vi "WinHostTocRIO.vi"() -> ()   [LabVIEW 2013]
uses:
  <vilib>/userdefined/High Color/nirio_resource_hc.ctl
  <vilib>/nisyscfg/Find Hardware.vi
  <vilib>/nisyscfg/Close (System).vi
  <vilib>/FPGAPlugInAG/NI 9159/niLvFpga_Open_NI 9159.vi
  <vilib>/rvi/interface/common/dynamic/niFpgaDynamicAddResources.vi
  <vilib>/rvi/interface/common/niFpgaWaitOnOcc.vi
  <vilib>/Utility/error.llb/Error Cluster From Error Code.vi
  <vilib>/FPGAPlugInAG/Dynamic/niLvFpga_Reset_Dynamic.vi
  <vilib>/FPGAPlugInAG/Dynamic/niLvFpga_Run_Dynamic.vi
  <vilib>/rvi/errors/niLvFpgaAdjustHostInterfaceError.vi
  <vilib>/FPGAPlugInAG/Dynamic/niLvFpga_Close_Dynamic.vi
  <vilib>/rvi/interface/nirviOpenFPGA/nirviOpenFPGA.xnode
  FPGA Bitfiles/cRIO9159_cRIODAQDMA_v1_1.lvbitx
  <vilib>/rvi/interface/nirviMethod/nirviMethod.xnode
  <vilib>/rvi/interface/nirviReadWriteControl/nirviReadWriteControl.xnode
  <vilib>/rvi/interface/nirviCloseFPGA/nirviCloseFPGA.xnode
  <vilib>/rvi/interface/Simulation/niFpgaSimulationCallBeginRW.vi
  <vilib>/rvi/errors/niLvFpgaMergeErrorWithErrorCode.vi
  <vilib>/FPGAPlugInAG/Dynamic/niLvFpga_ReadFifo_Dynamic.vi
  NiFpgaLv.dll
  <vilib>/nisyscfg/nisyscfg.lvlib
  <resource>/objmgr/nisysapi.rc
  <vilib>/FPGAPlugInAG/Dynamic/niLvFpga_ConfigureFifo_Dynamic.vi
  <vilib>/FPGAPlugInAG/Dynamic/niLvFpga_StartFifo_Dynamic.vi
  <vilib>/FPGAPlugInAG/Dynamic/niLvFpga_StopFifo_Dynamic.vi
panel:
  in  "stop":bool
  out "resource name":T1
  out "Resource":string="RIO0"
  out "resources out":refnum<k20>[](array[refnum])
  out "Waveform Graph":waveform(dbl)[](graph)
  out "error out":errorcluster
  out "Elements Remaining 3":u32
  out "Elements Remaining 2":u32
  in  "Tab Control":T2(tab)
  out "FPGAVIversion":u8[](array[numeric])=[1, 0]
  out "InsertedIOModulesID":u16[](array[numeric]) format="%x"
  out "InitDone":bool
  out "cRIOModulesOK":bool
  in  "DebugMode":bool
  out "DevQualityStatus":u8
  out "DeviceTemp":sgl format="%#1.2f"
  in  "DAQStartStop":bool
  out "DevProfile":u8
  out "Fref":u32
  out "DMATtoHOSTNCh":u16[](array[numeric])=[2]
  out "DMATtoHOSTFrameType":u8[](array[numeric])
  out "DMATtoHOSTSampleSize":u8[](array[numeric])=[4]
  out "DMATtoHOSTBlockNWords":u16[](array[numeric])=[128]
  out "DMATtoHOSTSamplingRate0":u16=1
  out "Elements Remaining":u32
  out "*(type *) &x":i32[](array[numeric])=[-730742, -4984294, -731430, -7767672, -730742, -9796516, -730053, -10862915, -730742, -10864292, -730053, -9799269, -730053, -7779375, -730742, -4991867, -730053, -1712809, -730742, 1728033, -730053, 5007779, -730742, 7793223, -730742, 9820002, -731430, 10887778, -730053, 10889843, -730742, 9825509, -731430, 7804238, -730742, 5014664, -730742, 1735606, -730053, -1705236, -730742, -4985671, -730053, -7766983, -731430, -9796516, -730053, -10861538, -731430, -10864292, -731430, -9799269, -729365, -7777999, -730742, -4991867, -731430, -1712809, -730053, 1727345, -730053, 5007779, -730053, 7791846, -730742, 9820690, -730742, 10887089, -732119, 10889843, -730742, 9824821, -730742, 7804238, -730742, 5013287, -730742, 1734229, -730053, -1705236, -730053, -4984982, -730053, -7766983, -730742, -9796516, -730053, -10862227, -730053, -10863604, -730742, -9799269, -730742, -7780064, -730053, -4991178, -731430, -1713497, -730742, 1726656, -730742, 5007091, -732119, 7792535, -730053, 9820002, -730742, 10887778, -730053, 10887089, -730053, 9824132, -730053, 7804238, -730742, 5014664, -730742, 1734918, -730742, -1705236, -732119, -4983605, -730742, -7766983, -730742, -9795827, -730053, -10862227, -730053, -10864292, -730742, -9799269, -730742, -7778687, -730742, -4990490, -730053, -1713497, -730742, 1728033, -731430, 5007779, -730742, 7791846, -731430, 9820690, -730053, 10887089, -731430, 10888466, -731430, 9824821, -730742, 7804238, -730053, 5013975, -730053, 1736295, -730053, -1704547, -732119, -4983605, -731430, -7766295, -730053, -9795139, -730742, -10861538, -730742, -10862915, -730053, -9798581, -730742, -7778687, -730742, -4991178, -731430, -1712809, -730742, 1725968, -731430, 5007779, -730053, 7791158, -732119, 9820002, -730742, 10887089, -730742, 10888466, -731430, 9824132, -730053, 7805615, -730742, 5015352, -730742, 1736295, -730742, -1704547, -730742, -4983605, -730742, -7766983, -729365, -9795827, -731430, -10862227, -730742, -10863604, -730053, -9800646, -730053, -7779375, -731430, -4991867, -731430, -1712809, -730053, 1726656, -731430, 5007091, -729365, 7792535, -730742, 9820690, -731430, 10887778, -731430, 10888466, -730742, 9824132, -730742, 7804927, -730742, 5014664, -731430, 1736295, -731430, -1702482, -730742, -4983605, -730742, -7766295, -730742, -9795139, -730053, -10862227, -730742, -10864292, -730742, -9799269, -730053, -7780752, -730742, -4992555] format="%x"
  out "Array":fxp<+/-,26,5>[](array[numeric])=[-0.34844493865966797, -2.3766965866088867, -0.3487730026245117, -3.7039146423339844, -0.34844493865966797, -4.671342849731445, -0.348116397857666, -5.1798415184021, -0.34844493865966797, -5.180498123168945, -0.348116397857666, -4.6726555824279785, -0.348116397857666, -3.7094950675964355, -0.34844493865966797, -2.380307674407959, -0.348116397857666, -0.8167309761047363, -0.34844493865966797, 0.8239903450012207, -0.348116397857666, 2.387895107269287, -0.34844493865966797, 3.7160983085632324, -0.34844493865966797, 4.682541847229004, -0.3487730026245117, 5.191697120666504, -0.348116397857666, 5.192681789398193, -0.34844493865966797, 4.6851677894592285, -0.3487730026245117, 3.72135066986084, -0.34844493865966797, 2.3911781311035156, -0.34844493865966797, 0.827601432800293, -0.348116397857666, -0.8131198883056641, -0.34844493865966797, -2.3773531913757324, -0.348116397857666, -3.7035861015319824, -0.3487730026245117, -4.671342849731445, -0.348116397857666, -5.179184913635254, -0.3487730026245117, -5.180498123168945, -0.3487730026245117, -4.6726555824279785, -0.34778833389282227, -3.708838939666748, -0.34844493865966797, -2.380307674407959, -0.3487730026245117, -0.8167309761047363, -0.348116397857666, 0.823662281036377, -0.348116397857666, 2.387895107269287, -0.348116397857666, 3.7154417037963867, -0.34844493865966797, 4.682869911193848, -0.34844493865966797, 5.191368579864502, -0.34910154342651367, 5.192681789398193, -0.34844493865966797, 4.684839725494385, -0.34844493865966797, 3.72135066986084, -0.34844493865966797, 2.39052152633667, -0.34844493865966797, 0.8269448280334473, -0.348116397857666, -0.8131198883056641, -0.348116397857666, -2.3770246505737305, -0.348116397857666, -3.7035861015319824, -0.34844493865966797, -4.671342849731445, -0.348116397857666, -5.179513454437256, -0.348116397857666, -5.180170059204102, -0.34844493865966797, -4.6726555824279785, -0.34844493865966797, -3.7098236083984375, -0.348116397857666, -2.379979133605957, -0.3487730026245117, -0.8170590400695801, -0.34844493865966797, 0.823333740234375, -0.34844493865966797, 2.3875670433044434, -0.34910154342651367, 3.7157702445983887, -0.348116397857666, 4.682541847229004, -0.34844493865966797, 5.191697120666504, -0.348116397857666, 5.191368579864502, -0.348116397857666, 4.684511184692383, -0.348116397857666, 3.72135066986084, -0.34844493865966797, 2.3911781311035156, -0.34844493865966797, 0.8272733688354492, -0.34844493865966797, -0.8131198883056641, -0.34910154342651367, -2.3763680458068848, -0.34844493865966797, -3.7035861015319824, -0.34844493865966797, -4.671014308929443, -0.348116397857666, -5.179513454437256, -0.348116397857666, -5.180498123168945, -0.34844493865966797, -4.6726555824279785, -0.34844493865966797, -3.709167003631592, -0.34844493865966797, -2.3796510696411133, -0.348116397857666, -0.8170590400695801, -0.34844493865966797, 0.8239903450012207, -0.3487730026245117, 2.387895107269287, -0.34844493865966797, 3.7154417037963867, -0.3487730026245117, 4.682869911193848, -0.348116397857666, 5.191368579864502, -0.3487730026245117, 5.192025184631348, -0.3487730026245117, 4.684839725494385, -0.34844493865966797, 3.72135066986084, -0.348116397857666, 2.3908495903015137, -0.348116397857666, 0.8279299736022949, -0.348116397857666, -0.8127913475036621, -0.34910154342651367, -2.3763680458068848, -0.3487730026245117, -3.7032580375671387, -0.348116397857666, -4.6706862449646, -0.34844493865966797, -5.179184913635254, -0.34844493865966797, -5.1798415184021, -0.348116397857666, -4.672327518463135, -0.34844493865966797, -3.709167003631592, -0.34844493865966797, -2.379979133605957, -0.3487730026245117, -0.8167309761047363, -0.34844493865966797, 0.8230056762695312, -0.3487730026245117, 2.387895107269287, -0.348116397857666, 3.715113639831543, -0.34910154342651367, 4.682541847229004, -0.34844493865966797, 5.191368579864502, -0.34844493865966797, 5.192025184631348, -0.3487730026245117, 4.684511184692383, -0.348116397857666, 3.7220072746276855, -0.34844493865966797, 2.3915061950683594, -0.34844493865966797, 0.8279299736022949, -0.34844493865966797, -0.8127913475036621, -0.34844493865966797, -2.3763680458068848, -0.34844493865966797, -3.7035861015319824, -0.34778833389282227, -4.671014308929443, -0.3487730026245117, -5.179513454437256, -0.34844493865966797, -5.180170059204102, -0.348116397857666, -4.673312187194824, -0.348116397857666, -3.7094950675964355, -0.3487730026245117, -2.380307674407959, -0.3487730026245117, -0.8167309761047363, -0.348116397857666, 0.823333740234375, -0.3487730026245117, 2.3875670433044434, -0.34778833389282227, 3.7157702445983887, -0.34844493865966797, 4.682869911193848, -0.3487730026245117, 5.191697120666504, -0.3487730026245117, 5.192025184631348, -0.34844493865966797, 4.684511184692383, -0.34844493865966797, 3.721679210662842, -0.34844493865966797, 2.3911781311035156, -0.3487730026245117, 0.8279299736022949, -0.3487730026245117, -0.8118066787719727, -0.34844493865966797, -2.3763680458068848, -0.34844493865966797, -3.7032580375671387, -0.34844493865966797, -4.6706862449646, -0.348116397857666, -5.179513454437256, -0.34844493865966797, -5.180498123168945, -0.34844493865966797, -4.6726555824279785, -0.348116397857666, -3.7101516723632812, -0.34844493865966797, -2.3806357383728027]
  out "Data":u64[](array[numeric])=[18443605565007720986, 18443602610067437960, 18443605565002908764, 18443608524234309309, 18443605565001840988, 18443608524235372955, 18443608524237392849, 18443605565007713413, 18443608524243459415, 18443605560719466017, 18443608519955212707, 18443605560725531207, 18443605560727557986, 18443602605791126114, 18443608519961094771, 18443605560727563493, 18443602605788042574, 18443605560722752648, 18443605560719473590, 18443608524243466988, 18443605565007719609, 18443608524237405241, 18443602610065409116, 18443608524234310686, 18443602610064341340, 18443602610065406363, 18443611479174893873, 18443605565007713413, 18443602610073492823, 18443608519951932273, 18443608519955212707, 18443608519957996774, 18443605560727558674, 18443605560728625073, 18443599646558661235, 18443605560727562805, 18443605560725542222, 18443605560722751271, 18443605560719472213, 18443608524243466988, 18443608524240187242, 18443608524237405241, 18443605565002908764, 18443608524234309997, 18443608524234308620, 18443605565002906011, 18443605565004925216, 18443608524240181046, 18443602610073492135, 18443605560719464640, 18443605560722745075, 18443599646555563927, 18443608519960024930, 18443605560728625762, 18443608519961092017, 18443608519960029060, 18443608519958009166, 18443605560722752648, 18443605560719472902, 18443605565011000044, 18443599650837755083, 18443605565004938297, 18443605565002909453, 18443608524234309997, 18443608524234307932, 18443605565002906011, 18443605565004926593, 18443605565007714790, 18443608524243458727, 18443605560719466017, 18443602605785246115, 18443605560725529830, 18443602605790059026, 18443608519961092017, 18443602605791126802, 18443602605790063157, 18443605560725542222, 18443608519955218903, 18443608519951941223, 18443608524243467677, 18443599650837755083, 18443602610067439337, 18443608524235377085, 18443605565001843742, 18443605565001842365, 18443608524235373643, 18443605565004926593, 18443605565007714102, 18443602610073492823, 18443605560719463952, 18443602605785246115, 18443608519957996086, 18443599646557591394, 18443605560728625073, 18443605560728626450, 18443602605790062468, 18443608519958010543, 18443605560722753336, 18443605560719474279, 18443605565011000733, 18443605565007721675, 18443605565004938297, 18443611479172876045, 18443602610064343405, 18443605565001841676, 18443608524235371578, 18443608524237392849, 18443602610070213765, 18443602610073492823, 18443608519951931584, 18443602605785245427, 18443611474895497111, 18443605560727558674, 18443602605791126114, 18443602605791126802, 18443605560727562116, 18443605560725542911, 18443605560722752648, 18443602605781974631, 18443602610073503150, 18443605565007721675, 18443605565004938985, 18443605565002910141, 18443608524234309997, 18443605565001840988, 18443605565002906011, 18443608524237391472, 18443605565007712725]
  in  "AO0":fxp<+/-,20,5>
  in  "AO1":fxp<+/-,20,5>
  in  "SGSignalType0":u8=1 max=3
  in  "SGPhase0":u32
  out "SGAmp0":u16
  in  "SGFreq0":sgl=50.0
  in  "SGAmp0":fxp<+/-,20,5>
  in  "SGUpdateRate0":u32=50
  out "AI1":fxp<+/-,26,5>
  out "AI0":fxp<+/-,26,5>
  in  "AOEnable0":bool
  in  "AOEnable1":bool
  out "AI2":fxp<+/-,26,5>
  in  "AO2":fxp<+/-,20,5>
  in  "AOEnable2":bool
  out "SGFref0":u32
  in  "Desired Sampling Rate":dbl=1000.0 max=1000.0
  out "SamplingRate":dbl
  in  "DO0":bool
  in  "DO1":bool
  in  "DO2":bool
  in  "auxDO1":bool
  out "DI0":bool
  out "DI1":bool
  out "DI2":bool
  out "auxDI1":bool
  out "Numeric":i32
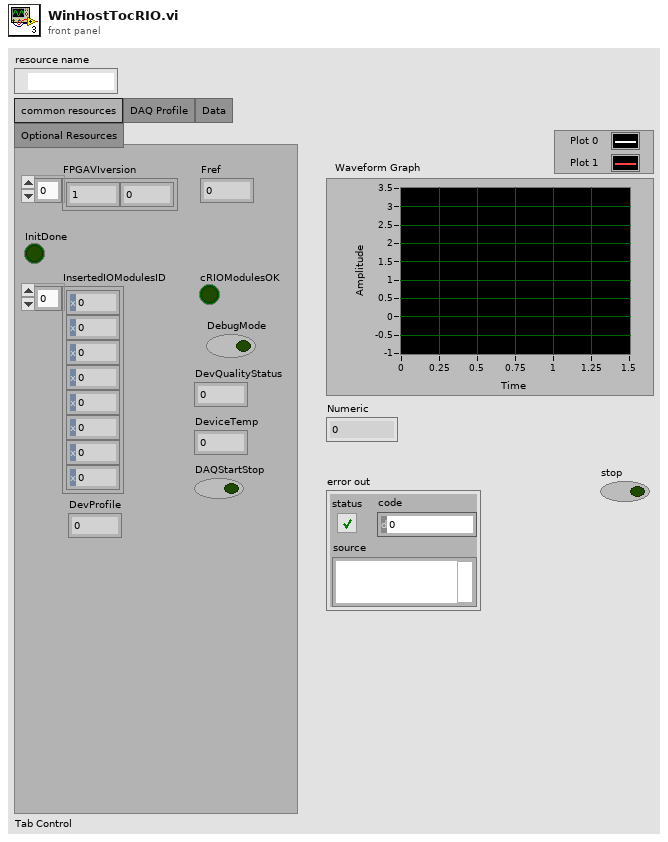
[diagram p1: front panel]
types:
  T1 = typedef "nirio_resource_hc.ctl" = tag
  T2 = enum32{"common resources", "DAQ Profile", "Data", "Optional Resources"}
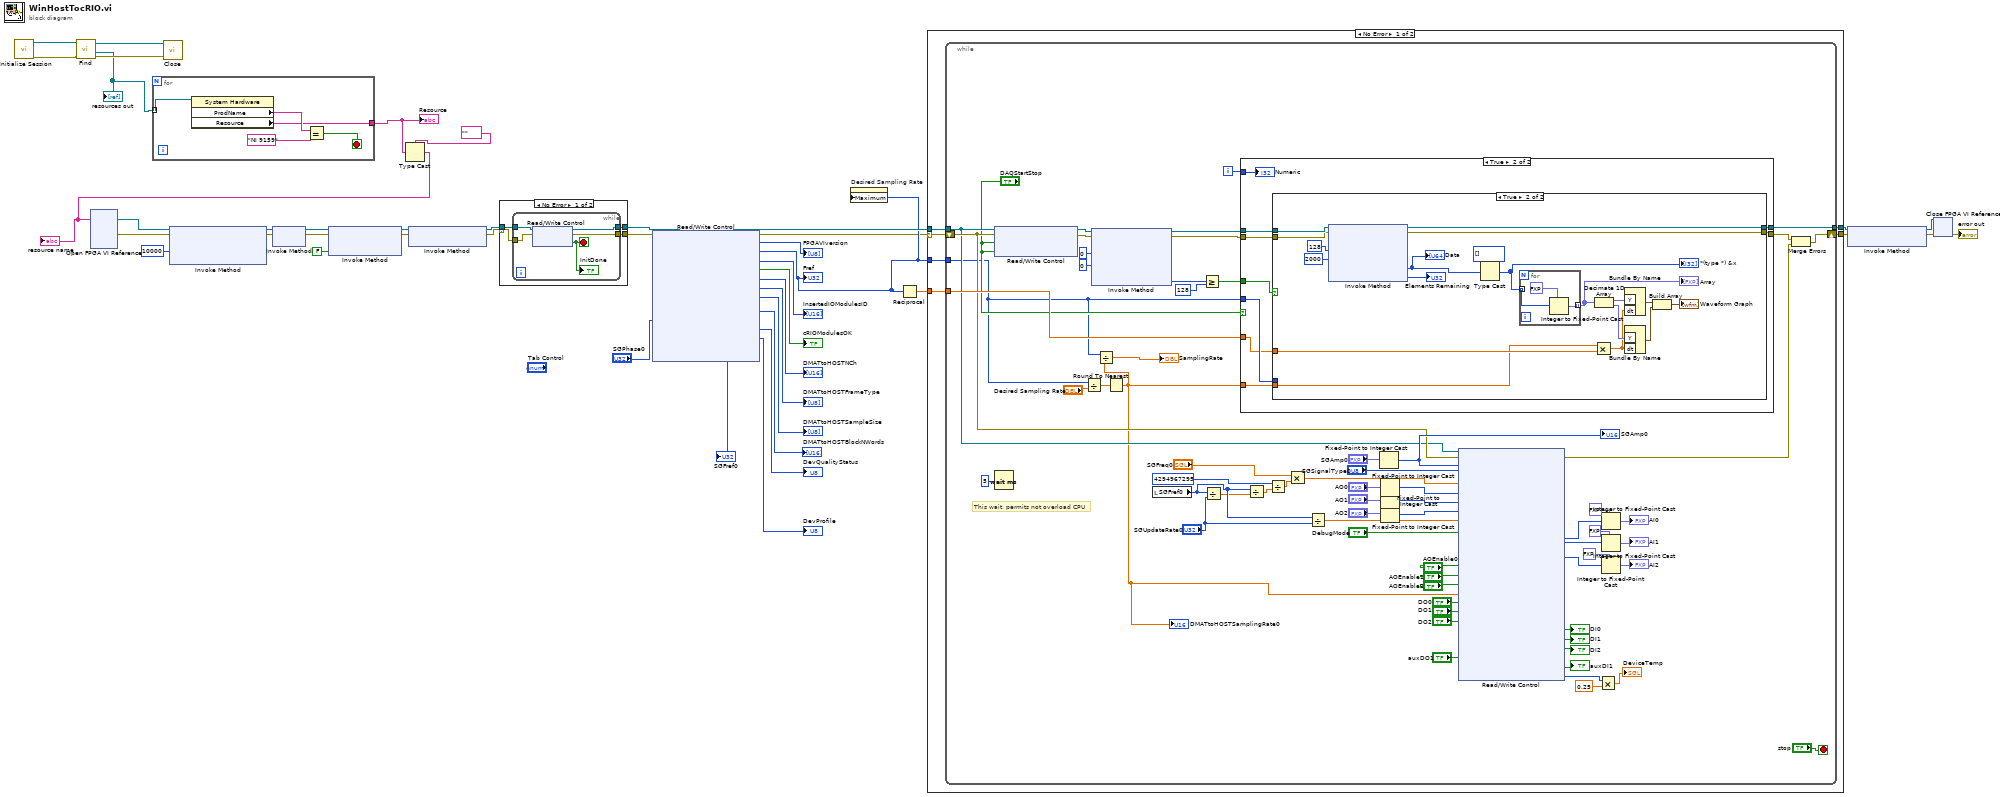
[diagram p0: block diagram]
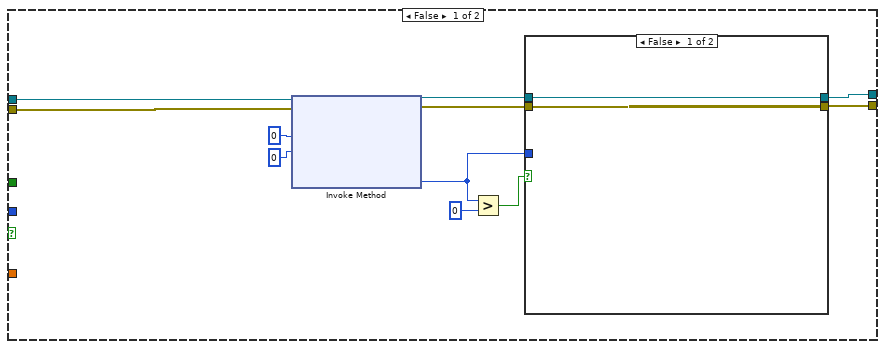
[diagram p2: hidden frame]
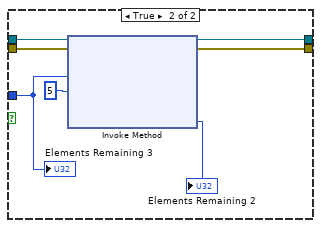
[diagram p3: hidden frame]
diagram:
  n1 = call <vilib>:"Initialize Session.vi"() -> ("error out"=w7:errorcluster, "session out"=w8:refnum<k21>)  [unwired: 10 in]
  n2 = call-poly <vilib>:"Find.vi"("error in (no error)"=w7, "session in"=w8) -> ("error out"=w5:errorcluster, "resources out"=w4:refnum<k20>[], "session out"=w6:refnum<k21>)  [unwired: 6 in, 1 out]
  "resources out" <- w4
  n3 = for {
    tunnel: w4 -> [w47] mode=indexing
    tunnel: [w43] -> w3
    stop <- w44 stop-if-true
    n4 = property class="System Hardware"(reference=w47) -> ("ProdName"=w45:string, "Resource"=w43:string)  [unwired: 1 in, 2 out]
    n5 = Equal?(x=w45, y="NI 9159") -> (x = y?=w44:bool)
  }
  "Resource" <- w3
  n6 = call-poly <vilib>:"Close.vi"("error in (no error)"=w5, "session in"=w6) -> ()  [unwired: 9 in, 1 out]
  n7 = Type Cast(type=T1 "" ("resource name 2"), x=w3) -> (*(type *) &x=w1:T1)
  "resource name" <- w1
  n8 = xnode "Open FPGA VI Reference"("resource name"=w1) -> ("FPGA VI Reference Out"=w30:refnum<k20>, "error out"=w29:errorcluster)  [unwired: 1 in]
  n9 = xnode "Invoke Method"("FPGA VI Reference In"=w30, "error in"=w29, "Requested Depth"=u32 10000) -> ("FPGA VI Reference Out"=w28:refnum<k20>, "error out"=w27:errorcluster)  [unwired: 1 out]
  n10 = xnode "Invoke Method"("FPGA VI Reference In"=w28, "error in"=w27) -> ("FPGA VI Reference Out"=w42:refnum<k20>, "error out"=w41:errorcluster)
  n11 = xnode "Invoke Method"("FPGA VI Reference In"=w42, "error in"=w41, "Wait Until Done (F)"=FALSE) -> ("FPGA VI Reference Out"=w25:refnum<k20>, "error out"=w24:errorcluster)
  n12 = xnode "Invoke Method"("FPGA VI Reference In"=w25, "error in"=w24) -> ("FPGA VI Reference Out"=w23:refnum<k20>, "error out"=w11:errorcluster)
  n13 = case shown="No Error" w11 {
    selector: w11 -> [w48 w58]
    tunnel: [w51 w57] -> w38
    tunnel: [w50 w58] -> w37
    tunnel: w23 -> [w49 w57]
    frame No Error {
      n14 = while {
        tunnel: w49 -> [w56]
        tunnel: [w54] -> w51
        tunnel: [w53] -> w50
        tunnel: w48 -> [w52]
        stop <- w55 stop-if-true
        n15 = xnode "Read/Write Control"("FPGA VI Reference In"=w56, "error in"=w52) -> ("FPGA VI Reference Out"=w54:refnum<k20>, "error out"=w53:errorcluster, "InitDone"=w55:bool)
        "InitDone" <- w55
      }
    }
    frame Error {
    }
  }
  n16 = xnode "Read/Write Control"("FPGA VI Reference In"=w38, "error in"=w37, "SGPhase0"="SGPhase0") -> ("FPGA VI Reference Out"=w31:refnum<k20>, "error out"=w10:errorcluster, "FPGAVIversion"=→"FPGAVIversion":u8[], "Fref"=w13:u32, "InsertedIOModulesID"=→"InsertedIOModulesID":u16[], "cRIOModulesOK"=→"cRIOModulesOK":bool, "DMATtoHOSTNCh"=→"DMATtoHOSTNCh":u16[], "DMATtoHOSTFrameType"=→"DMATtoHOSTFrameType":u8[], "DMATtoHOSTSampleSize"=→"DMATtoHOSTSampleSize":u8[], "DMATtoHOSTBlockNWords"=→"DMATtoHOSTBlockNWords":u16[], "DevQualityStatus"=→"DevQualityStatus":u8, "DevProfile"=→"DevProfile":u8, "SGFref0"=→"SGFref0":u32)  [unwired: 1 in]
  "Fref" <- w13
  n17 = property on="Desired Sampling Rate" class="DigNum (strict)"("Maximum"=w13) -> ()  [unwired: 2 in, 2 out]
  n18 = Reciprocal(x=w13) -> (1/x=w14:dbl)
  n19 = case shown="No Error" w10 {
    selector: w10 -> [w59 w186]
    tunnel: w31 -> [w64 w185]
    tunnel: [w63 w185] -> w22
    tunnel: [w62 w186] -> w21
    tunnel: w14 -> [w61 _]
    tunnel: w13 -> [w60 _]
    frame No Error {
      n20 = while {
        tunnel: w64 -> [w79]
        tunnel: [w130] -> w63
        tunnel: w61 -> [w128]
        tunnel: w60 -> [w66]
        shift-right: [w81] -> w62
        shift-left: w59 -> [w80]
        i -> [w129]
        stop <- "stop" stop-if-true
        # "This wait, permits not overload CPU"
        n21 = xnode "Read/Write Control"("FPGA VI Reference In"=w79, "error in"=w80, "DMATtoHOSTEnable0"="DAQStartStop", "DAQStartStop"="DAQStartStop") -> ("FPGA VI Reference Out"=w77:refnum<k20>, "error out"=w76:errorcluster)
        n22 = Wait (ms)(milliseconds to wait=u32 5) -> ()  [unwired: 1 out]
        n23 = Divide(x=w66, y="Desired Sampling Rate") -> (x/y=w85:dbl)
        n24 = xnode "Invoke Method"("FPGA VI Reference In"=w77, "error in"=w76, "Number of Elements"=u32 0, "Timeout (ms)"=0) -> ("FPGA VI Reference Out"=w72:refnum<k20>, "error out"=w71:errorcluster, "Elements Remaining"=w75:u32)  [unwired: 1 out]
        n25 = Round To Nearest(number=w85) -> (nearest integer value=w65:dbl)
        "DMATtoHOSTSamplingRate0" <- w65
        n26 = Divide(x=w66, y=w65) -> (x/y=→"SamplingRate":dbl)
        n27 = local read "SGFref0"() -> (w116:u32)
        n28 = Greater Or Equal?(x=w75, y=u32 128) -> (x >= y?=w70:bool)
        n29 = Divide(x=w116, y="SGUpdateRate0") -> (x/y=w105:dbl)
        n30 = case shown="True" "DAQStartStop" {
          tunnel: [w138 w152] -> w130
          tunnel: [w137 w156] -> w83
          tunnel: w129 -> [_ w160]
          tunnel: w128 -> [_ w158]
          tunnel: w66 -> [_ w159]
          tunnel: w65 -> [_ w157]
          tunnel: w72 -> [w133 w154]
          tunnel: w71 -> [w132 w153]
          tunnel: w70 -> [_ w155]
          frame False {
            n31 = xnode "Invoke Method"("FPGA VI Reference In"=w133, "error in"=w132, "Number of Elements"=u32 0, "Timeout (ms)"=0) -> ("FPGA VI Reference Out"=w140:refnum<k20>, "error out"=w139:errorcluster, "Elements Remaining"=w134:u32)  [unwired: 1 out]
            n32 = Greater?(x=w134, y=u32 0) -> (0:w135:bool)
            n33 = case shown="False" w135 {
              tunnel: w140 -> [w144 w151]
              tunnel: w139 -> [w143 w150]
              tunnel: [w144 w147] -> w138
              tunnel: [w143 w146] -> w137
              tunnel: w134 -> [_ w145]
              frame False {
              }
              frame True {
                n34 = xnode "Invoke Method"("FPGA VI Reference In"=w151, "error in"=w150, "Number of Elements"=w145, "Timeout (ms)"=5) -> ("FPGA VI Reference Out"=w147:refnum<k20>, "error out"=w146:errorcluster, "Elements Remaining"=→"Elements Remaining 2":u32)  [unwired: 1 out]
                "Elements Remaining 3" <- w145
              }
            }
          }
          frame True {
            n35 = case shown="True" w155 {
              tunnel: w159 -> [_ _]
              tunnel: w158 -> [_ w169]
              tunnel: w157 -> [_ w168]
              tunnel: [w161 w166] -> w156
              tunnel: w154 -> [w162 w165]
              tunnel: w153 -> [w161 w164]
              tunnel: [w162 w163] -> w152
              frame False {
              }
              frame True {
                n36 = xnode "Invoke Method"("FPGA VI Reference In"=w165, "error in"=w164, "Number of Elements"=u32 128, "Timeout (ms)"=2000) -> ("FPGA VI Reference Out"=w163:refnum<k20>, "error out"=w166:errorcluster, "Data"=w179:u64[], "Elements Remaining"=→"Elements Remaining":u32)
                "Data" <- w179
                n37 = Type Cast(type=i32[] [], x=w179) -> (*(type *) &x=w177:i32[])
                "*(type *) &x" <- w177
                n38 = for {
                  tunnel: w177 -> [w184] mode=indexing
                  tunnel: [w183] -> w176 mode=indexing
                  n39 = Integer to Fixed-Point Cast(fixed-point type=fxp<+/-,26,5> 0.0, integer=w184) -> (fixed-point=w183:fxp<+/-,26,5>)
                }
                "Array" <- w176
                n40 = Multiply(x=w168, y=w169) -> (x*y=w171:dbl)
                n41 = Decimate 1D Array(w176) -> (w175:fxp<+/-,26,5>[], w173:fxp<+/-,26,5>[])
                n42 = Bundle By Name("Y"=w175, "dt"=w171) -> (w174:waveform(dbl))  [unwired: 1 in]
                n43 = Bundle By Name("Y"=w173, "dt"=w171) -> (w172:waveform(dbl))  [unwired: 1 in]
                n44 = Build Array(w174, w172) -> (→"Waveform Graph":waveform(dbl)[])
              }
            }
            "Numeric" <- w160
          }
        }
        n45 = Divide(x=w116, y=w105) -> (x/y=w107:dbl)
        n46 = Divide(x=i64 4294967295, y=w107) -> (x/y=w108:dbl)
        n47 = Multiply(x="SGFreq0", y=w108) -> (x*y=w109:dbl)
        n48 = Divide(x=w116, y="SGUpdateRate0") -> (x/y=w94:dbl)
        n49 = Fixed-Point to Integer Cast(1:"SGAmp0") -> (0:w93:i32)
        "SGAmp0" <- w93
        n50 = Fixed-Point to Integer Cast(1:"AO0") -> (0:w89:i32)
        n51 = Fixed-Point to Integer Cast(1:"AO1") -> (0:w91:i32)
        n52 = Fixed-Point to Integer Cast(1:"AO2") -> (0:w115:i32)
        n53 = xnode "Read/Write Control"("FPGA VI Reference In"=w79, "error in"=w80, "SGAmp0"=w93, "SGSignalType0"="SGSignalType0", "SGFreq0"=w109, "AO0"=w89, "AO1"=w91, "AO2"=w115, "SGUpdateRate0"=w94, "DebugMode"="DebugMode", "AOEnable0"="AOEnable0", "AOEnable1"="AOEnable1", "AOEnable2"="AOEnable2", "DMATtoHOSTSamplingRate0"=w65, "DO0"="DO0", "DO1"="DO1", "DO2"="DO2", "auxDO0"="auxDO1") -> ("error out"=w82:errorcluster, "AI0"=w111:i32, "AI1"=w113:i32, "AI2"=w114:i32, "DI0"=→"DI0":bool, "DI1"=→"DI1":bool, "DI2"=→"DI2":bool, "auxDI0"=→"auxDI1":bool, "DevTemp"=w126:i16)  [unwired: 1 out]
        n54 = Multiply(x=w126, y=sgl 0.25) -> (x*y=→"DeviceTemp":sgl)
        n55 = Integer to Fixed-Point Cast(fixed-point type=fxp<+/-,26,5> 0.0, integer=w111) -> (fixed-point=→"AI0":fxp<+/-,26,5>)
        n56 = Integer to Fixed-Point Cast(fixed-point type=fxp<+/-,26,5> 0.0, integer=w113) -> (fixed-point=→"AI1":fxp<+/-,26,5>)
        n57 = Integer to Fixed-Point Cast(fixed-point type=fxp<+/-,26,5> 0.0, integer=w114) -> (fixed-point=→"AI2":fxp<+/-,26,5>)
        n58 = Merge Errors(w83, w82) -> (w81:errorcluster)
      }
    }
    frame Error {
    }
  }
  n59 = xnode "Invoke Method"("FPGA VI Reference In"=w22, "error in"=w21) -> ("FPGA VI Reference Out"=w20:refnum<k20>, "error out"=w19:errorcluster)
  n60 = xnode "Close FPGA VI Reference"("FPGA VI Reference In"=w20, "error in"=w19) -> ("error out"=→"error out":errorcluster)
